vi "GetDependencies.vi"(8 "error in (no error)":errorcluster, 11 "SubVI in":refnum<vi>) -> (0 "error out":errorcluster, 1 "Dependency Paths":path[](array[path]), 2 "Dependency Names":string[](array[string]), 3 "SubVI out":refnum<vi>)   [LabVIEW 2017]
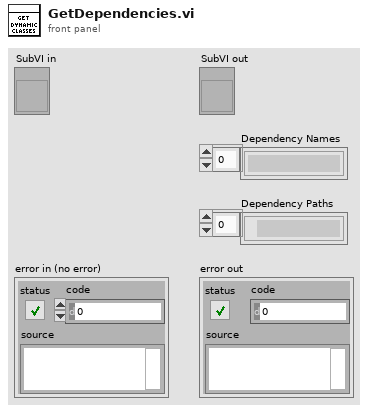
[diagram p1: front panel]
types:
  T1 = enum8{"No dynamic dispatch VIs", "Include nearest implementation", "Include all overrides"}
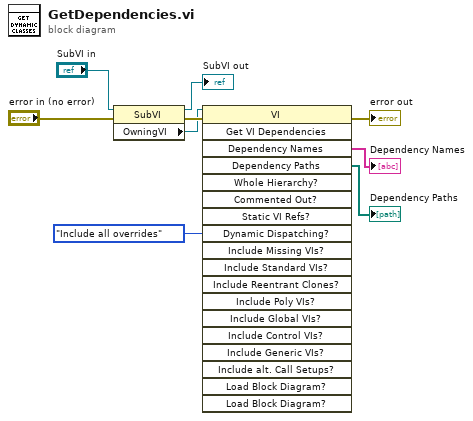
[diagram p0: block diagram]
diagram:
  n1 = property class="SubVI"(reference="SubVI in", error in="error in (no error)") -> (reference out=→"SubVI out":refnum<vi>, error out=w5:errorcluster, "OwningVI"=w3:refnum<vi>)
  n2 = invoke class="VI" method="Get VI Dependencies"(reference=w3, error in=w5, "Dynamic Dispatching?"=T1."Include all overrides") -> (error out=→"error out":errorcluster, "Dependency Names"=→"Dependency Names":string[], "Dependency Paths"=→"Dependency Paths":path[])  [unwired: 16 in, 16 out]
